vi "Task Monitoring.vi"() -> ()   [LabVIEW 2020]
panel:
  in  "Stop":bool
  out "Memory Usage History":sgl(graph)
  out "Memory Usage":sgl
  out "error out":errorcluster
  in  "stop":bool
  out "CPU Usage (%)":sgl(slide) scale=0.0..100.0
  out "Processor History":sgl(graph)
  out "cpu usage":sgl
  out "System Status":string
  in  "STOP VI":bool
  in  "IP Address to Ping":string="0.0.0.0"
  out "IP Free?":bool
  in  "PING IP":bool
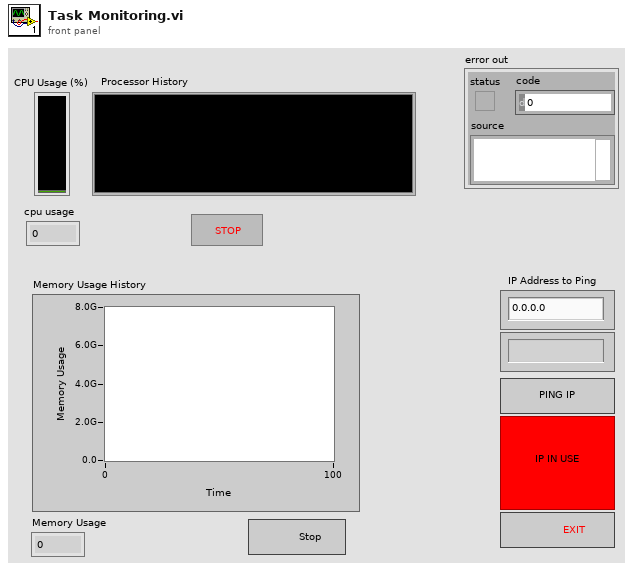
[diagram p1: front panel]
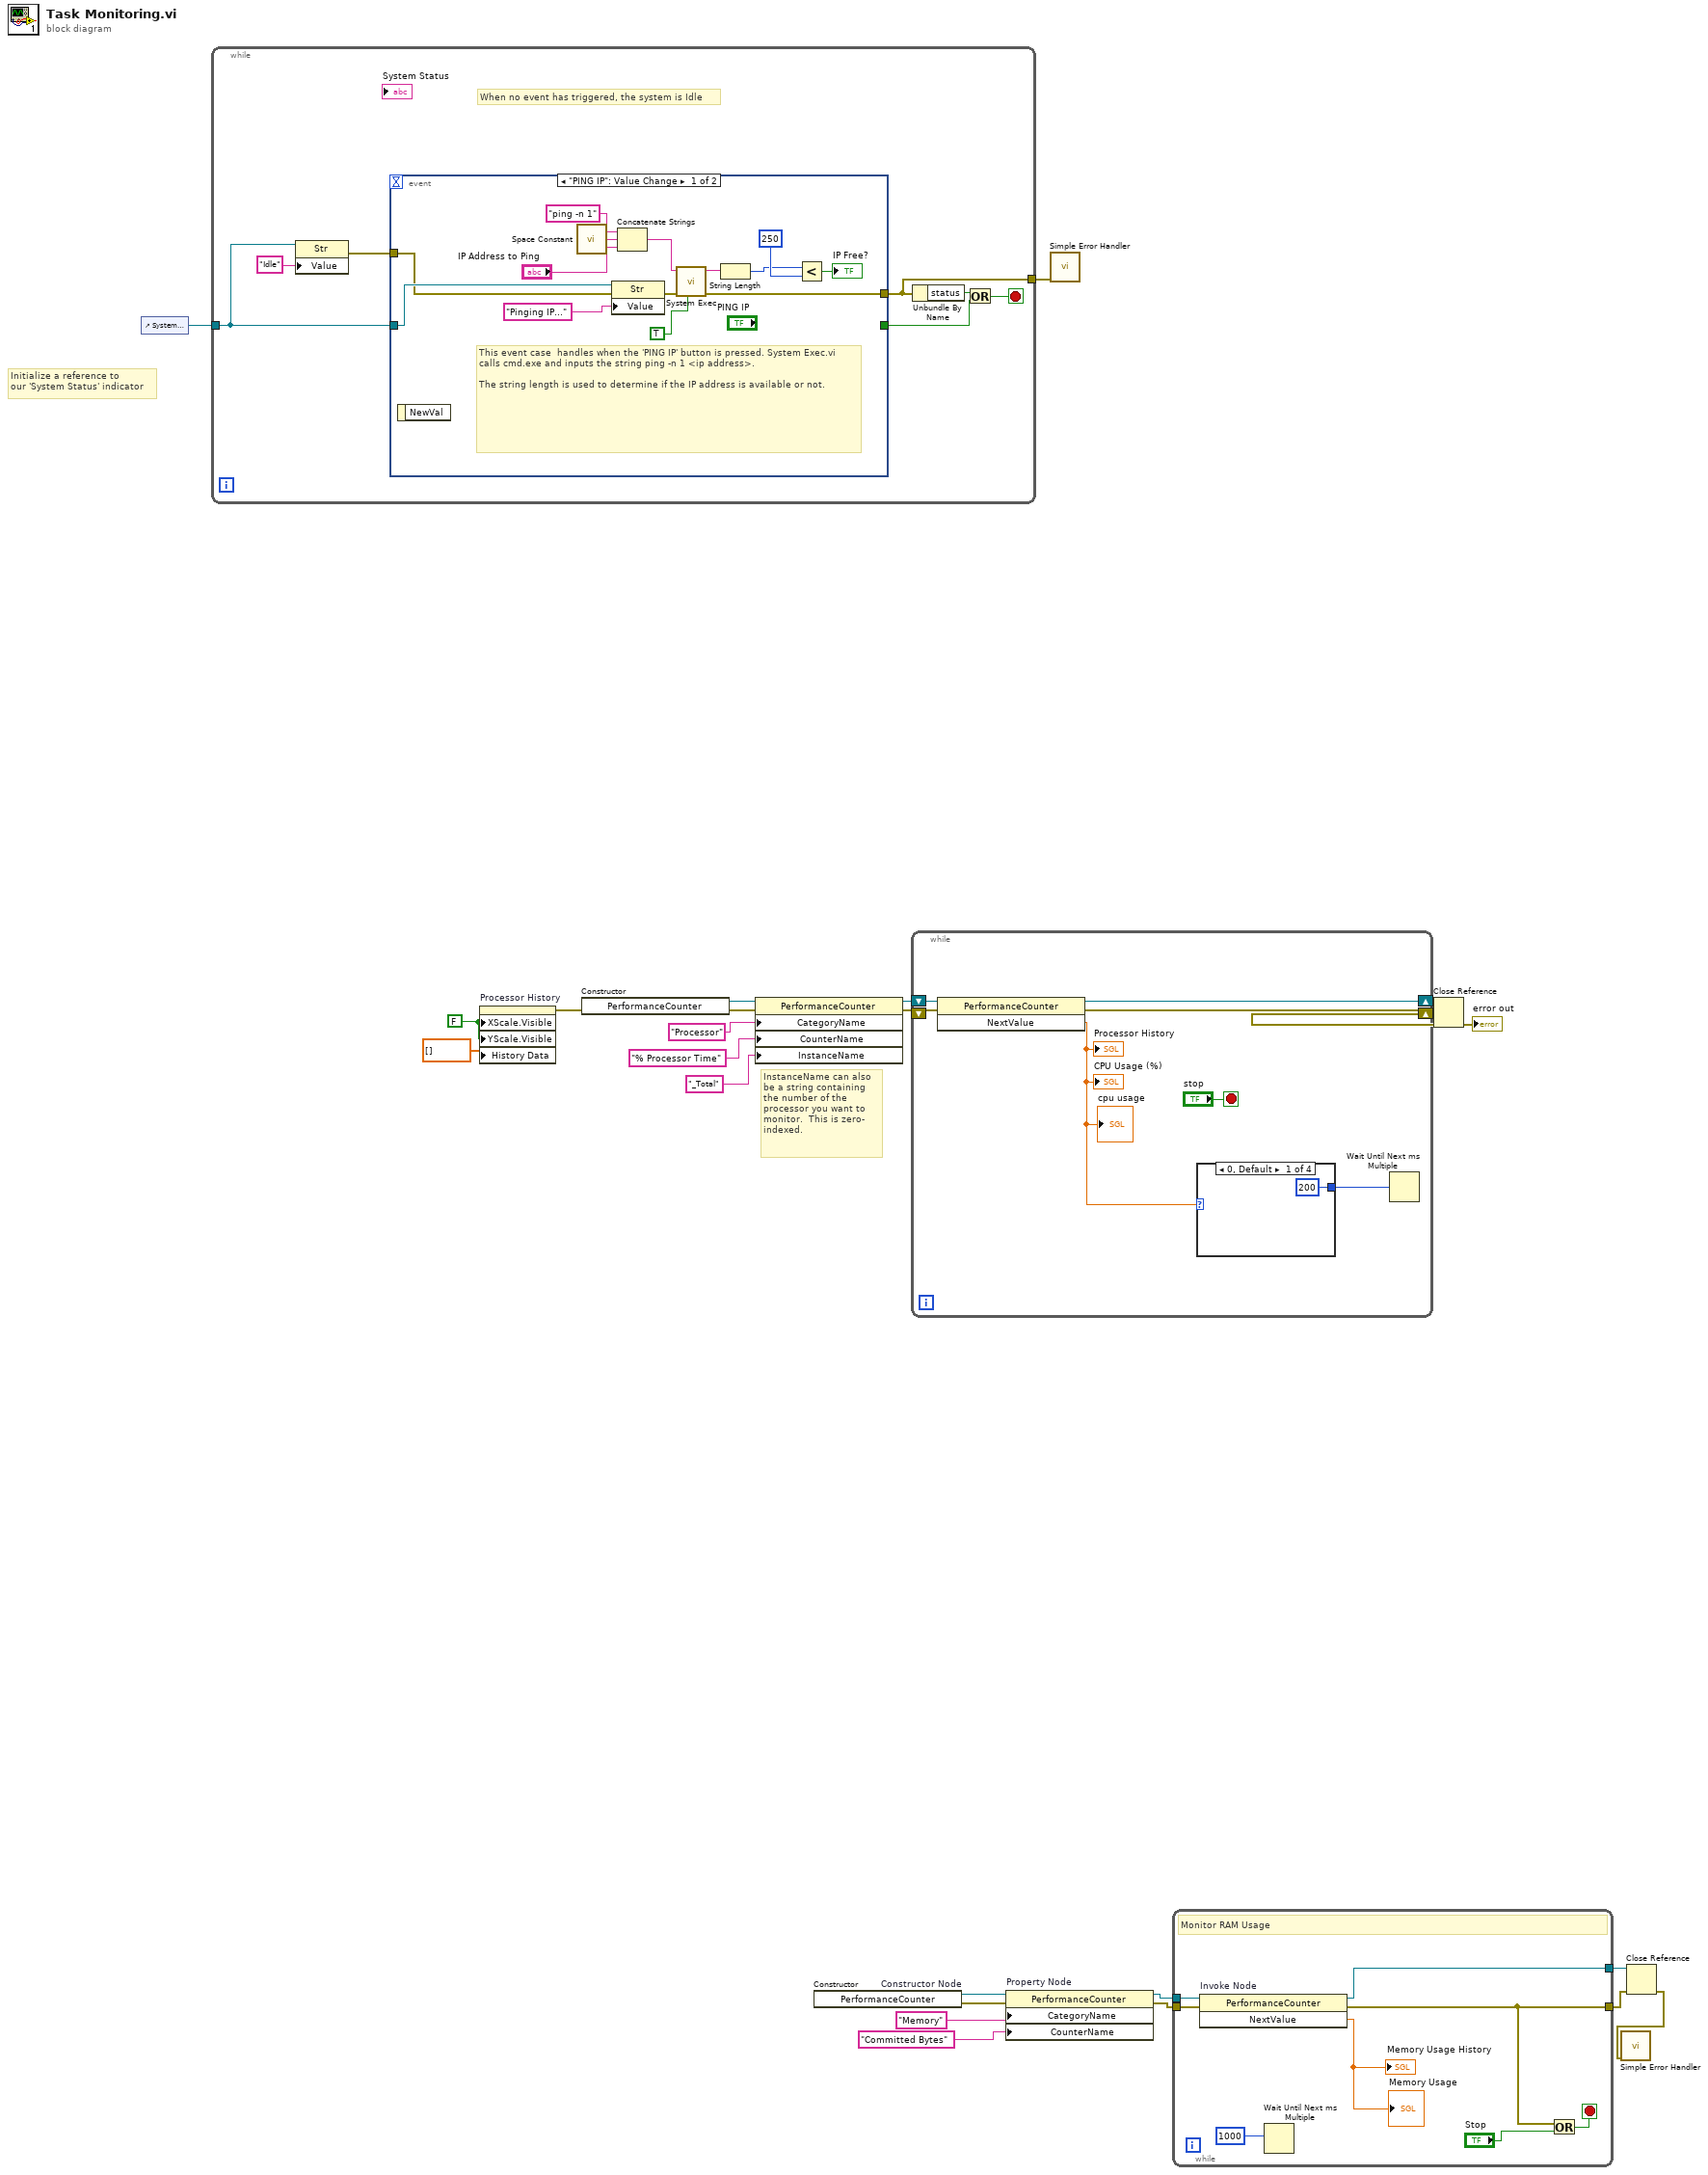
[diagram p0: block diagram]
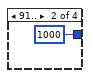
[diagram p2: hidden frame]
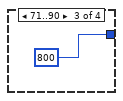
[diagram p3: hidden frame]
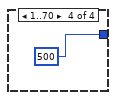
[diagram p4: hidden frame]
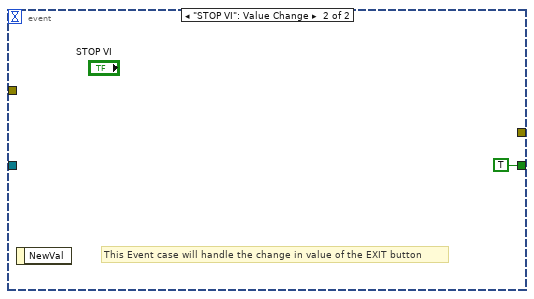
[diagram p5: hidden frame]
diagram:
  w13 = FALSE ("X Scale.Visible")
  # "InstanceName can also\nbe a string containing\nthe number of the\nprocessor you want to\nmonitor.  This is zero-\nindexed."
  # "Initialize a reference to\nour 'System Status' indicator"
  n1 = control-ref of="System Status"() -> (w23:refnum<vi>)
  n2 = while {
    tunnel: [w31] -> w24
    tunnel: w23 -> [w27]
    stop <- w26 stop-if-true
    # "When no event has triggered, the system is Idle"
    n3 = property class="Str"(reference=w27, "Value"="Idle" ("System Status")) -> (error out=w25:errorcluster)  [unwired: 1 in, 1 out]
    n4 = event shown="[0] \"PING IP\": Value Change" {
      selector: _ -> [_ _]
      dyn-events: _ -> [_ _]
      timeout: _ -> [_ _]
      tunnel: [w45 _] -> w31
      tunnel: [_ TRUE] -> w29
      tunnel: w27 -> [w36 _]
      tunnel: w25 -> [w33 _]
      event "PING IP": Value Change {
        # "This event case  handles when the 'PING IP' button is pressed. System Exec.vi calls cmd.exe and inputs the string ping -n 1 <ip address>.\n\nThe string length is used to determine if the IP address is available or not."
        n5 = event-data() -> ()  [unwired: 1 in, 1 out]
        n6 = call <vilib>:"Space Constant.vi"() -> ("String"=w38:string)
        n7 = property class="Str"(reference=w36, error in=w33, "Value"="Pinging IP..." ("System Status")) -> (error out=w35:errorcluster)  [unwired: 1 out]
        n8 = Concatenate Strings("ping -n 1", w38, "IP Address to Ping") -> (w40:string)
        n9 = call <vilib>:"System Exec.vi"("run minimized? (F)"=TRUE, "error in (no error)"=w35, "command line"=w40) -> ("error out"=w45:errorcluster, "standard output"=w41:string)  [unwired: 5 in, 2 out]
        n10 = String Length(string=w41) -> (length=w42:i32)
        n11 = Less?(x=w42, y=250) -> (x < y?=→"IP Free?":bool)
      }
      event "STOP VI": Value Change {
        # "This Event case will handle the change in value of the EXIT button"
        n12 = event-data() -> ()  [unwired: 1 in, 1 out]
      }
    }
    n13 = Unbundle By Name(w31) -> ("status"=w30:bool)
    n14 = Or(x=w30, y=w29) -> (x .or. y?=w26:bool)
  }
  n15 = property on="Processor History" class="WFChart (strict)"("XScale.Visible"=w13, "YScale.Visible"=w13, "History Data"=sgl[] []) -> (error out=w10:errorcluster)  [unwired: 2 in, 1 out]
  n16 = constructor class="PerformanceCounter" ("Constructor Node")(error in=w10) -> (reference out=w22:refnum<k24>, error out=w21:errorcluster)  [unwired: 2 in, 1 out]
  n17 = property on="Property Node" class="PerformanceCounter"(reference=w22, error in=w21, "CategoryName"="Processor", "CounterName"="% Processor Time", "InstanceName"="_Total") -> (reference out=w18:refnum<k24>, error out=w17:errorcluster)
  n18 = constructor on="Constructor Node" class="PerformanceCounter"() -> (reference out=w6:refnum<k24>, error out=w5:errorcluster)  [unwired: 3 in, 1 out]
  n19 = while {
    shift-right: [w50] -> w15
    shift-left: w18 -> [w53]
    shift-right: [w51] -> w16
    shift-left: w17 -> [w52]
    stop <- "stop" stop-if-true
    n20 = invoke on="Invoke Node" class="PerformanceCounter" method="NextValue"(reference=w53, error in=w52) -> (reference out=w50:refnum<k24>, error out=w51:errorcluster, "NextValue"=w48:sgl)  [unwired: 1 in]
    "CPU Usage (%)" <- w48
    "Processor History" <- w48
    "cpu usage" <- w48
    n21 = case shown="0, Default" w48 {
      tunnel: [u32 200 ("milliseconds to wait") u32 1000 ("milliseconds to wait") u32 800 ("milliseconds to wait") u32 500 ("milliseconds to wait")] -> w47
      frame 0, Default {
      }
      frame 91.. {
      }
      frame 71..90 {
      }
      frame 1..70 {
      }
    }
    n22 = Wait Until Next ms Multiple(millisecond multiple=w47) -> ()  [unwired: 1 out]
  }
  n23 = property on="Property Node" class="PerformanceCounter"(reference=w6, error in=w5, "CategoryName"="Memory" ("categoryName"), "CounterName"="Committed Bytes" ("counterName")) -> (reference out=w4:refnum<k24>, error out=w3:errorcluster)
  n24 = call <vilib>:"Simple Error Handler.vi"("error in (no error)"=w24) -> ()  [unwired: 4 in, 5 out]
  n25 = while {
    tunnel: w4 -> [w63]
    tunnel: w3 -> [w62]
    tunnel: [w61] -> w9
    tunnel: [w60] -> w7
    stop <- w64 stop-if-true
    # "Monitor RAM Usage"
    n26 = invoke on="Invoke Node" class="PerformanceCounter" method="NextValue"(reference=w63, error in=w62) -> (reference out=w60:refnum<k24>, error out=w61:errorcluster, "NextValue"=→"Memory Usage History" →"Memory Usage":sgl)  [unwired: 1 in]
    n27 = Wait Until Next ms Multiple(millisecond multiple=u32 1000) -> ()  [unwired: 1 out]
    n28 = Or(x=w61, y="Stop") -> (x .or. y?=w64:bool)
  }
  n29 = Close Reference(reference=w15, error in (no error)=w16) -> (error out=→"error out":errorcluster)
  n30 = Close Reference(reference=w7, error in (no error)=w9) -> (error out=w8:errorcluster)
  n31 = call <vilib>:"Simple Error Handler.vi"("error in (no error)"=w8) -> ()  [unwired: 1 in, 8 out]
